vi "DmgrEnumDevices.vi"(8 "Error In":errorcluster) -> (0 "Error Out":errorcluster, 2 "Num Devices":i32)   [LabVIEW 2011, in "LVH-Adept.lvlib" / "DMGR.lvlib"]
doc: "Enumerate Devices"
uses:
  DMGR.lvlib
  Private/Type Defs/Error.ctl
  Resources/dmgr.dll
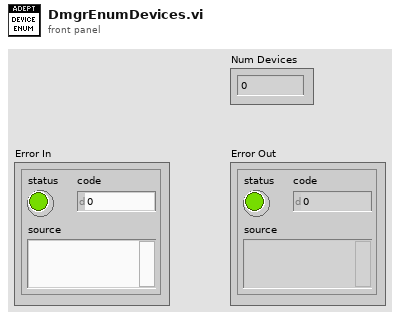
[diagram p1: front panel]
types:
  T1 = typedef "LVH-Adept.lvlib/DMGR.lvlib/Error.ctl" = enum16{"Unknown Error", "Device Enumeration", "Device Handle", "Device Info", "Device Open"}
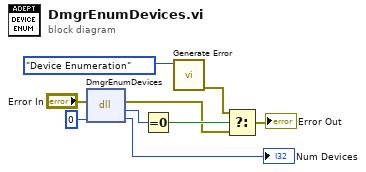
[diagram p0: block diagram]
diagram:
  n1 = dll-call lib="C:/github/makerhub/Adept/LabVIEW/vi.lib/MakerHub/Adept/Private/Resources/dmgr.dll" fn="DmgrEnumDevices"(error in="Error In", "pcdvc"=0) -> (error out=w2:errorcluster, "Error?"=w7:i8, "pcdvc"=→"Num Devices":i32)  [unwired: 2 in, 1 out]
  n2 = Equal To 0?(x=w7) -> (x = 0?=w6:bool)
  n3 = call "Generate Error.vi"("Error Type"=Error."Device Enumeration") -> ("Error Out"=w3:errorcluster)  [unwired: 10 in]
  n4 = Select(t=w3, s=w6, f=w2) -> (s? t:f=→"Error Out":errorcluster)
